vi "RelayAndDoTest.vi"(0 "类型":u32(ring)=4 items=["PCI5121"=1, "PCI9810"=2, "USBCAN1"=3, "USBCAN2"=4, "PCI9820"=5, "CAN232"=6, "PCI5110"=7, "CANLite(mini)"=8, "ISA9620"=9, "ISA5420"=10, "PC104CAN"=11, "CANET"=17, "DNP9810"=13, "USBCAN-E-U"=20, "USBCAN-2E-U"=21], 1 "设备索引":u32(ring) items=["0", "1", "2", "3", "4", "5", "6", "7", "8", "9", "10", "11", "12", "13", "14", "15", ""], 2 "功能":T1(ring), 3 "端口状态":enum16{"ON", "OFF"}(ring), 4 "CAN路数":u32(ring) items=["0", "1"]) -> (14 "发送成功?":bool)   [LabVIEW 2013]
panel:
  out "VCI_CAN_OBJ_T":T2 {"ID" format="%x"}
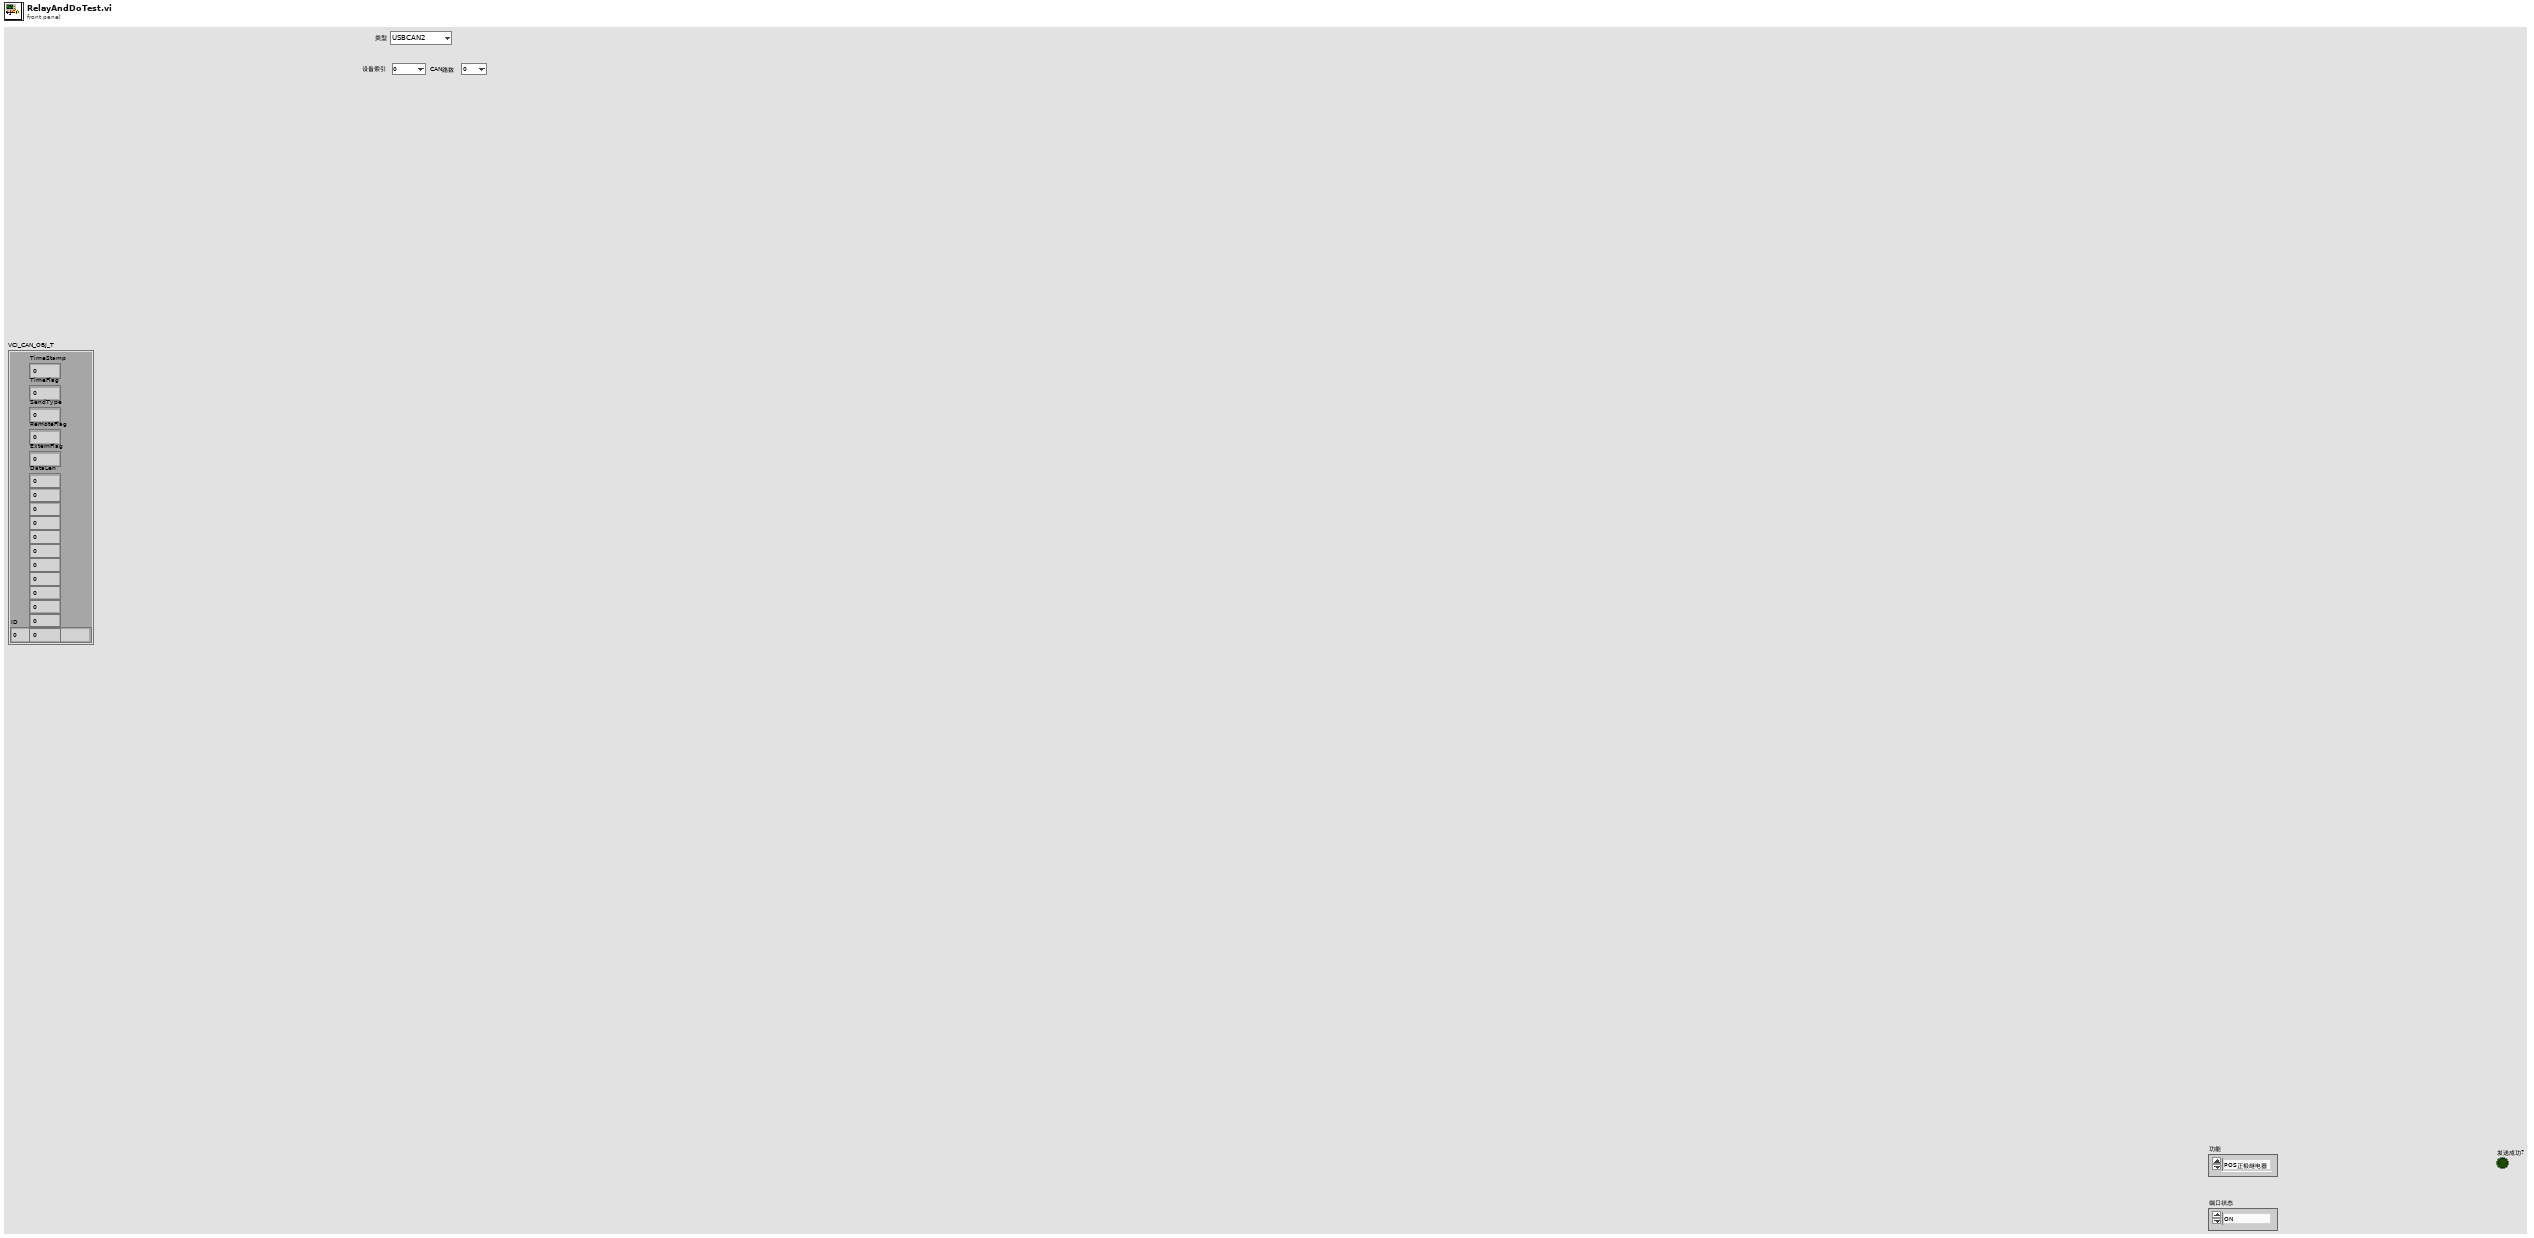
[diagram p1: front panel]
types:
  T1 = enum16{"POS正极继电器", "NEG负极继电器", "PRE预充继电器", "CHG充电继电器", "FAN风机继电器", "HEAT加热继电器", "DO1", "DO2"}
  T2 = cluster{"ID":u32, "TimeStamp":u32, "TimeFlag":u8, "SendType":u8, "RemoteFlag":u8, "ExternFlag":u8, "DataLen":u8, u8, u8, u8, u8, u8, u8, u8, u8, u8, u8, u8}
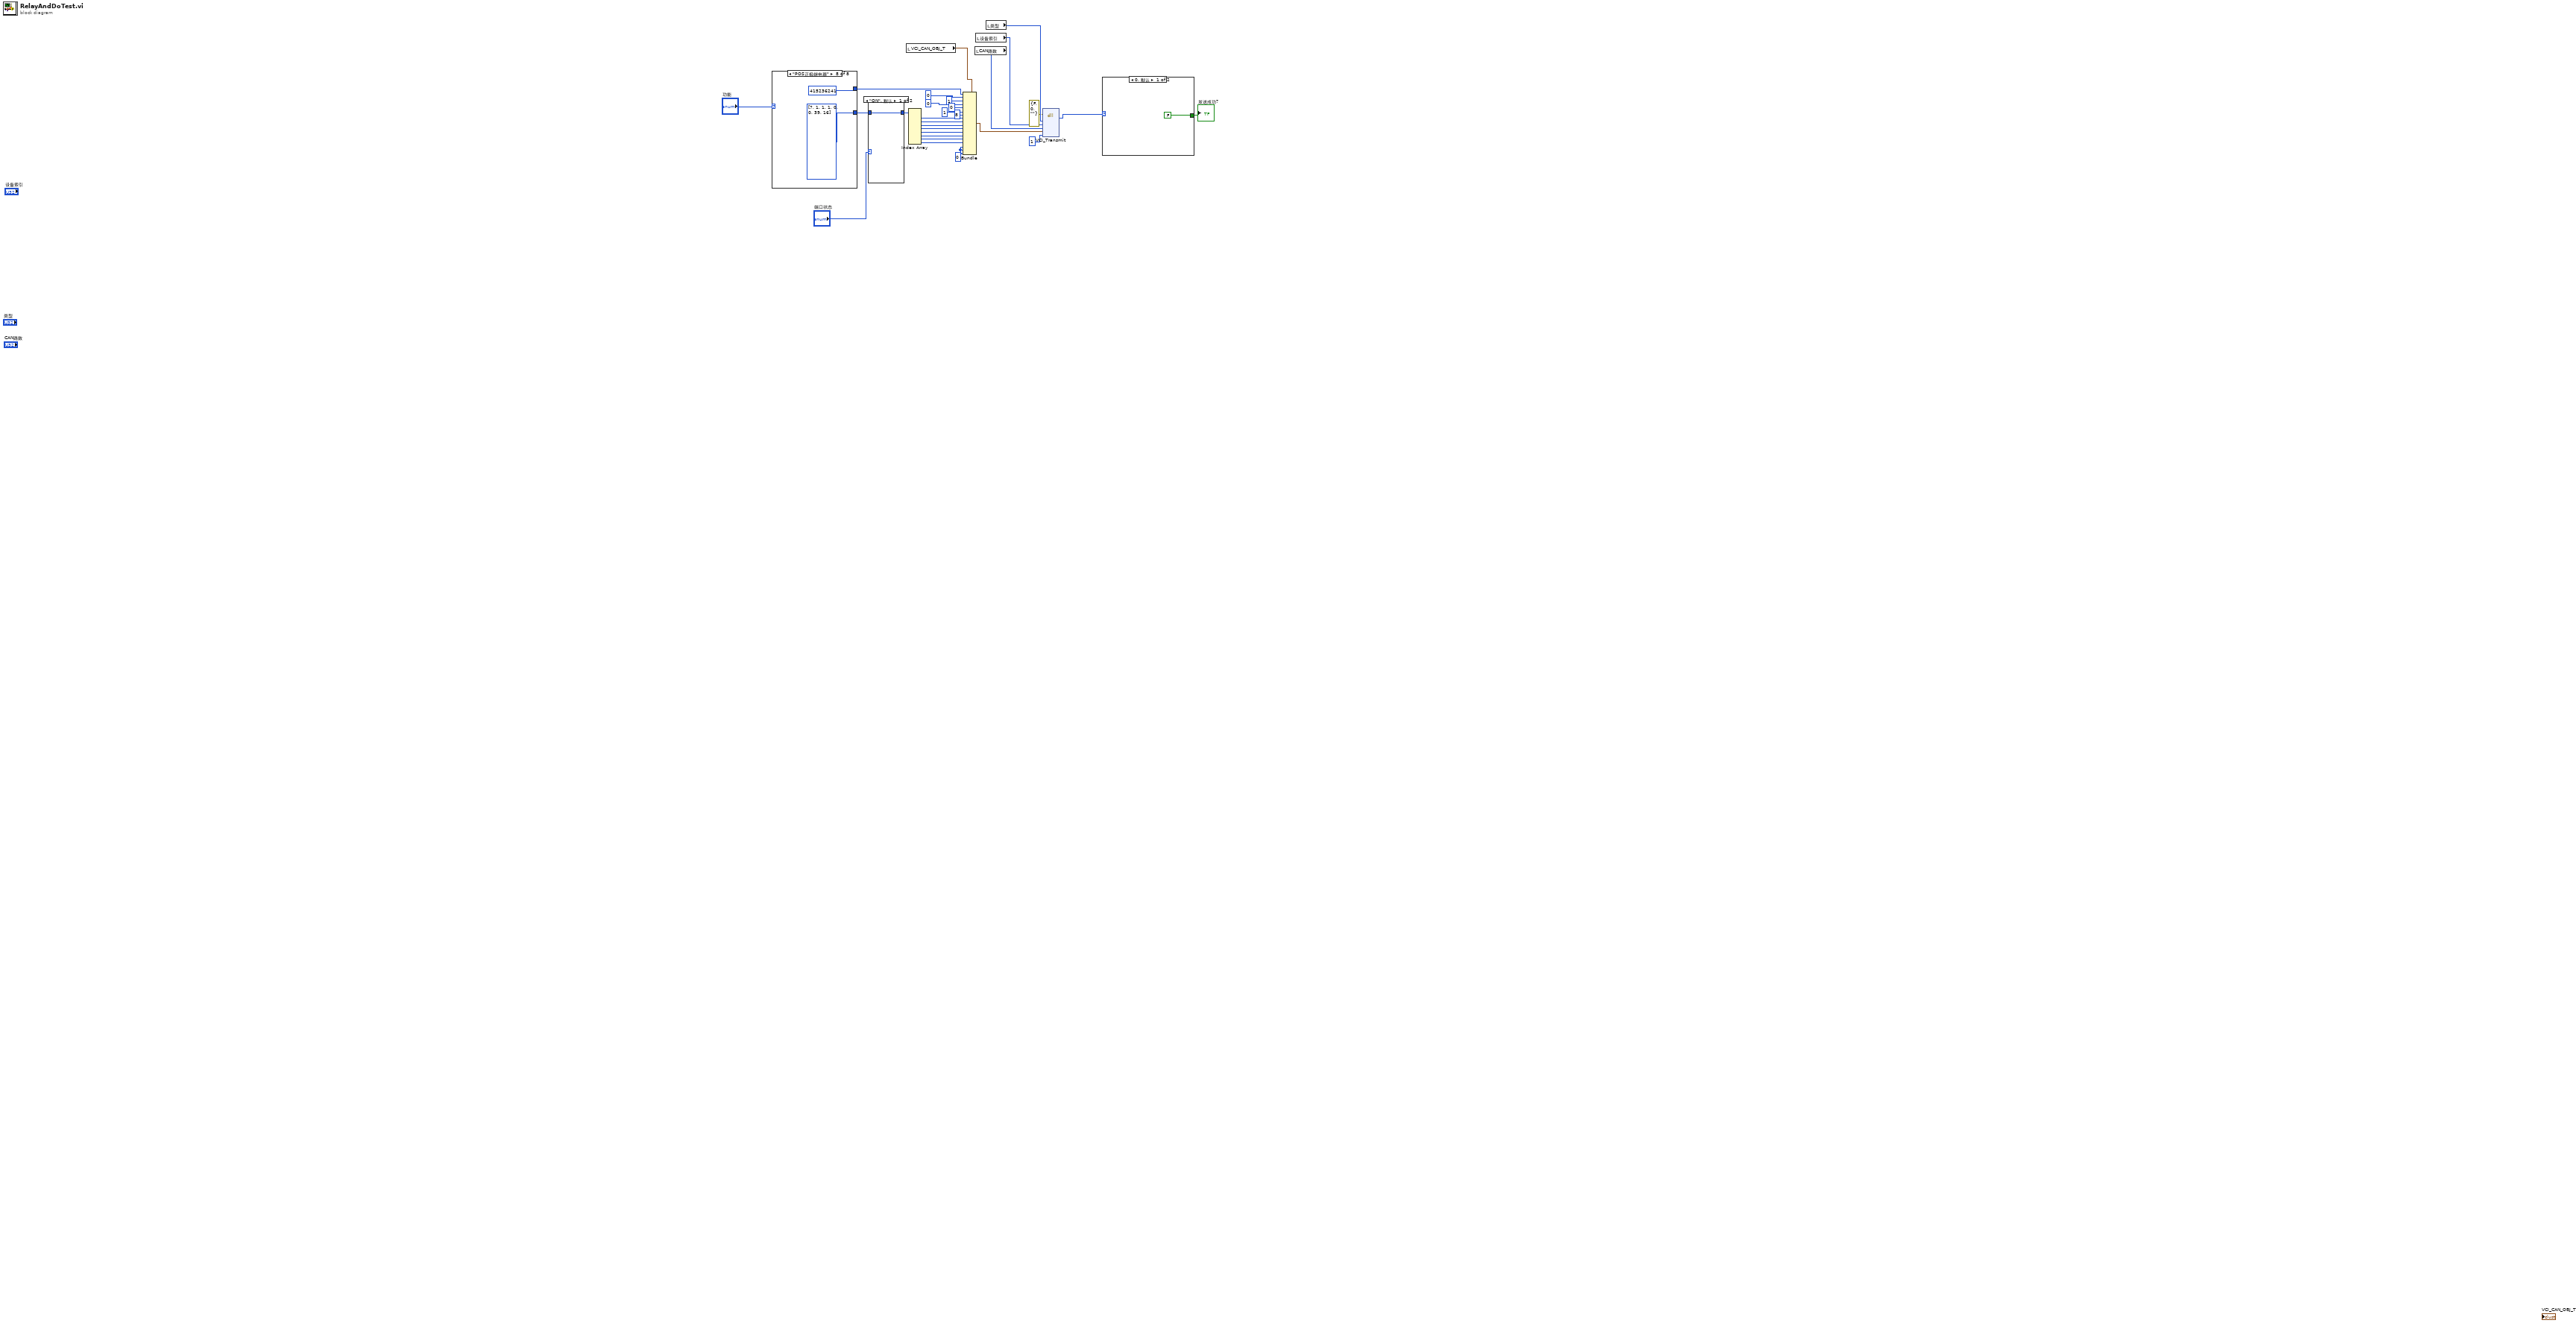
[diagram p0: block diagram]
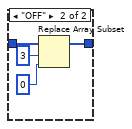
[diagram p2: hidden frame]
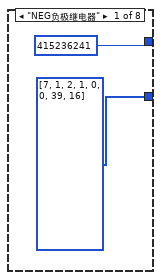
[diagram p3: hidden frame]
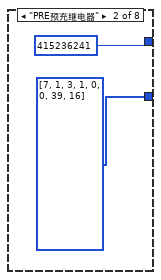
[diagram p4: hidden frame]
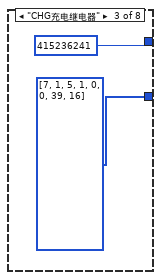
[diagram p5: hidden frame]
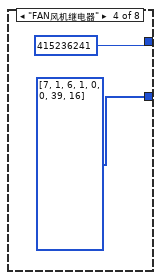
[diagram p6: hidden frame]
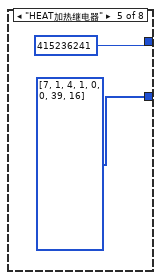
[diagram p7: hidden frame]
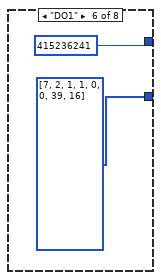
[diagram p8: hidden frame]
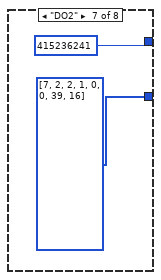
[diagram p9: hidden frame]
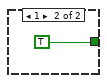
[diagram p10: hidden frame]
diagram:
  w20 = u8 0 ("元素")
  n1 = case shown="\"POS正极继电器\"" "功能" {
    tunnel: [u8[] [7, 1, 2, 1, 0, 0, 39, 16] ("数组") u8[] [7, 1, 3, 1, 0, 0, 39, 16] ("数组") u8[] [7, 1, 5, 1, 0, 0, 39, 16] ("数组") u8[] [7, 1, 6, 1, 0, 0, 39, 16] ("数组") u8[] [7, 1, 4, 1, 0, 0, 39, 16] ("数组") u8[] [7, 2, 1, 1, 0, 0, 39, 16] ("数组") u8[] [7, 2, 2, 1, 0, 0, 39, 16] ("数组") u8[] [7, 1, 1, 1, 0, 0, 39, 16] ("数组")] -> w2
    tunnel: [u32 415236241 ("RemoteFlag") u32 415236241 ("RemoteFlag") u32 415236241 ("RemoteFlag") u32 415236241 ("RemoteFlag") u32 415236241 ("RemoteFlag") u32 415236241 ("RemoteFlag") u32 415236241 ("RemoteFlag") u32 415236241 ("RemoteFlag")] -> w5
    frame "NEG负极继电器" {
    }
    frame "PRE预充继电器" {
    }
    frame "CHG充电继电器" {
    }
    frame "FAN风机继电器" {
    }
    frame "HEAT加热继电器" {
    }
    frame "DO1" {
    }
    frame "DO2" {
    }
    frame "POS正极继电器" {
    }
  }
  n2 = case shown="\"ON\", 默认" "端口状态" {
    tunnel: [w46 w49] -> w3
    tunnel: w2 -> [w46 w50]
    frame "ON", Default {
    }
    frame "OFF" {
      n3 = Replace Array Subset(array=w50, new element=u8 0 ("新元素/子数组"), index=3 ("索引")) -> (w49:u8[])
    }
  }
  n4 = local read "VCI_CAN_OBJ_T"() -> (w24:T2)
  n5 = Index Array(array=w3) -> (element #1=w18:u8, element #2=w17:u8, element #3=w16:u8, element #4=w15:u8, element #5=w14:u8, element #6=w13:u8, element #7=w12:u8, element #8=w11:u8)  [unwired: 8 in]
  n6 = Bundle(cluster=w24, "ID"=w5, "TimeStamp"=u8 0 ("RemoteFlag"), "TimeFlag"=u8 1, "SendType"=u8 0 ("DataLen"), "RemoteFlag"=u8 0, "ExternFlag"=u8 1, "DataLen"=u8 8, w18, w17, w16, w15, w14, w13, w12, w11, w20, w20, w20) -> (w28:T2)
  n7 = local read "CAN路数"() -> (w25:u32)
  n8 = local read "设备索引"() -> (w26:u32)
  n9 = local read "类型"() -> (w27:u32)
  n10 = dll-call lib="PTH1¦abs FBluewave New EnergySVN_WorkAutoTest_TestStandtrunkAutoTest_TestStandDriverZlgCanBHN01AutoBurnBMUåºç¨ç¨åºä¸..." fn="VCI_Transmit"(error in=errorcluster {"status"=FALSE, "code"=0, "source"=""} ("错误输入（无错误）"), "DeviceType"=w27, "DeviceInd"=w26, "CANInd"=w25, "pSend"=w28, "Len"=u32 1) -> ("返回类型"=w1:u32)  [unwired: 4 in, 5 out]
  n11 = case shown="0, 默认" w1 {
    tunnel: [FALSE TRUE] -> w9
    frame 0, Default {
    }
    frame 1 {
    }
  }
  "发送成功?" <- w9
